vi "power turn.vi"(9 "current angle":dbl, 11 "desired angle(degrees)":dbl) -> (2 "output":dbl)   [LabVIEW 2016]
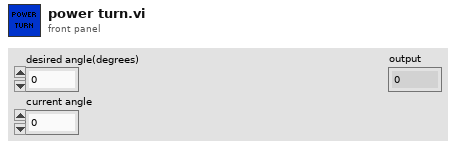
[diagram p1: front panel]
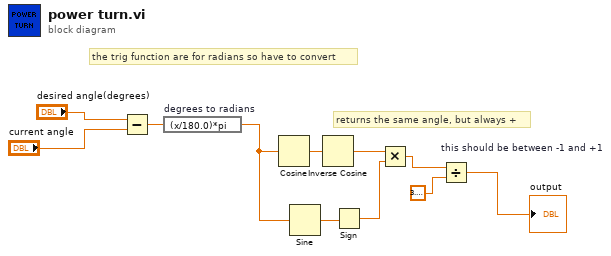
[diagram p0: block diagram]
diagram:
  # "returns the same angle, but always +"
  # "the trig function are for radians so have to convert"
  n1 = Subtract(x="desired angle(degrees)", y="current angle") -> (x-y=w9:dbl)
  n2 = expression code="(x/180.0)*pi" "degrees to radians"(w9) -> (w2:dbl)
  n3 = Cosine(x=w2) -> (cos(x)=w11:dbl)
  n4 = Sine(x=w2) -> (sin(x)=w10:dbl)
  n5 = Inverse Cosine(1:w11) -> (0:w8:dbl)
  n6 = Sign(1:w10) -> (0:w7:dbl)
  n7 = Multiply(x=w8, y=w7) -> (x*y=w6:dbl)
  n8 = Divide "this should be between -1 and +1"(x=w6, y=3.141592653589793) -> (x/y=→"output":dbl)
